vi "Process.vi"(8 "error in (no error)":errorcluster, 9 "Galvo.lvclass":refnum<class "Galvo.lvclass">, 10 "DAQ Class.lvclass":refnum<class "DAQ Class.lvclass">, 11 "Processing in":refnum<class "Processing.lvclass">) -> (0 "error out":errorcluster, 3 "Processing out":refnum<class "Processing.lvclass">)   [LabVIEW 2015, in "Processing.lvclass"]
uses:
  Processing.lvclass
  DAQ/DAQ Class.lvclass
  Galvo/Galvo.lvclass
  Processing.lvclass/Processing.ctl
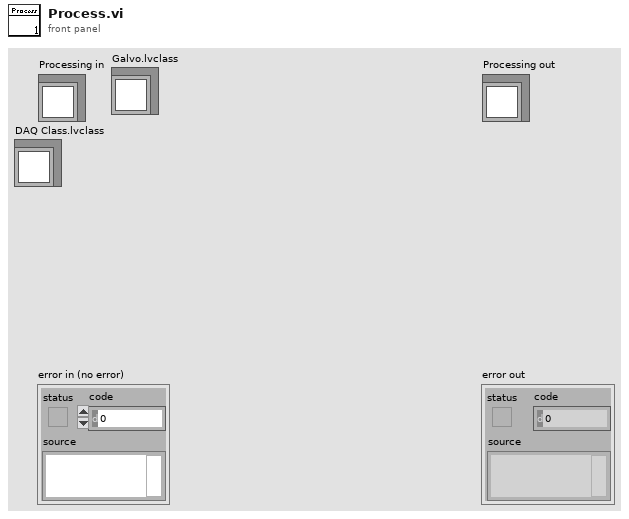
[diagram p1: front panel]
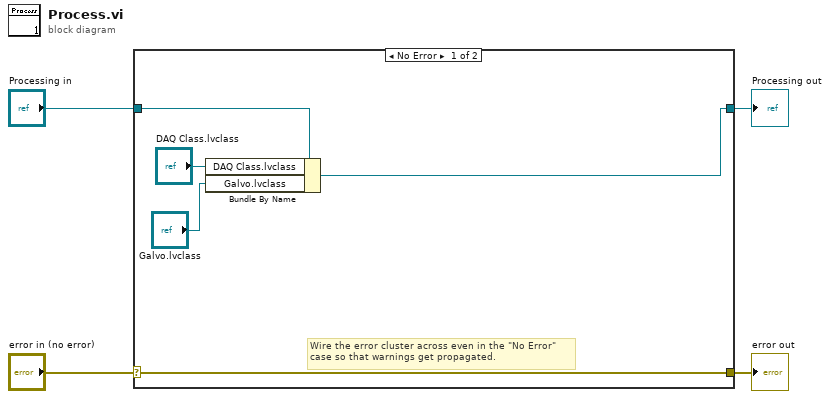
[diagram p0: block diagram]
diagram:
  n1 = case shown="No Error" "error in (no error)" {
    selector: "error in (no error)" -> [w9 w11]
    tunnel: [w9 w11] -> w3
    tunnel: [w7 w10] -> w1
    tunnel: "Processing in" -> [w8 w10]
    frame No Error {
      # "Wire the error cluster across even in the \"No Error\"\ncase so that warnings get propagated."
      n2 = Bundle By Name(cluster=w8, "DAQ Class.lvclass"="DAQ Class.lvclass", "Galvo.lvclass"="Galvo.lvclass") -> (w7:refnum<class "Processing.lvclass">)
    }
    frame Error {
    }
  }
  "error out" <- w3
  "Processing out" <- w1
